vi "Configure Systems.vi"() -> ()   [LabVIEW 2009, in "POLARIS BME DG.lvlib" / "BME_DG_System.lvclass"]
uses:
  DG Classes/BME_DG_System/BME_DG_System.lvclass
  DetectDG.ctl
  System DG Selection.ctl
  LV-BME Interface/BME_DG_TriggerSettings.ctl
  LV-BME Interface/ClockSource.ctl
  SG08_Settings.ctl
  LV-BME Interface/BME_DG_V2TriggerSettings.ctl
  MSBusSignals.ctl
  LV-BME Interface/ChnlSettings.ctl
  Go_Done_Chnl_Settings.ctl
  GoSignalBits.ctl
  SG08_Chnl_Settings.ctl
  Chnl Settings Complete.ctl
  Card Config.ctl
  <vilib>/Utility/xml.llb/Write to XML File(array).vi
  DG Classes/BME_DG_Chnl/BME_DG_Chnl.lvclass
  POLARIS BME DG.lvlib
panel:
  out "Error?":bool
  in  "Build System":bool
  in  "ChnlToSwap":u16(ring) items=["a", "b", "c", "d", "e", "f", "ma", "mb", "mc", "md", "me", "mf", "sa", "sb", "sc", "sd", "se", "sf"]
  in  "SwapChnlWith":bool
  in  "Card2":u16(ring) caption="Swap with" items=["Master", "Master of Slave", "Slave of Master"]
  in  "SwapCardsWith":bool
  in  "Stop search":bool=TRUE
  in  "Find Chnl":u16(ring) items=["a", "b", "c", "d", "e", "f", "ma", "mb", "mc", "md", "me", "mf", "sa", "sb", "sc", "sd", "se", "sf"]
  in  "Find Card":u16(ring) items=["Master", "Master of Slave", "Slave of Master"]
  in  "stop":bool
  in  "Tab Control":T1(tab)=enum."Check"
  in  "InstalledDGs":T2[](array[typedef])
  in  "Select System":u16(ring) items=["Einsamer Master", "Master and Servant"]
  in  "Systems":T3[](array[typedef])
  in  "Selected DG":u16(ring) items=["0", "1", "2"]
  in  "Add":bool
  in  "Remove":bool
  in  "Empty Systems":bool
  in  "DetectDGs":bool
  in  "Card Config":T9(array[cluster]) {"Advanced Settings"."Trigger on MS Bus" format="%04x" items=["Local Primary0x1"=1, "Local Secondary0x2"=2, "Local Force 0x4"=4, "Resynchronize 0x8"=8, "StepBackOnBus 0x10"=16, "StartOnBus 0x20"=32, "InhibitOnBus 0x40"=64, "LoadDataOnBus 0x80"=128]; "Advanced Settings"."Force Trigger (µs)" min=0.0 format="%.6f"; "SG08_Settings"."StepBackTime (µs)" min=0.0 format="%.6f"; "SG08_Settings"."Gate Delay (µs)" format="%.3f"; "SG08_Settings"."Gate Level" min=-2.5 max=2.5 format="%.3g"; "Base Settings"."Gate Divider" min=1 max=1000000; "Base Settings"."Clock Source" items=["Internal Oscillator"=1, "External Trigger"=2, "Trigger-> Oscillator"=3, "MasterSlave Bus"=4]; "Base Settings"."Inhibit(µs)" format="%#_11g"}
  in  "Copy Chnl\n Names":bool=TRUE
  in  "Chnls":T14(array[cluster]) {"ChnParameter"."Delay (µs)" min=0.0 max=100000000.0 format="%.4f"; "G08_Chnl_Settings"."Pulse Width (µs)" min=0.0 max=8947840.0 format="%#.6f"; "Go and Done Signal"."Done Signal" format="%04x" items=["Local Primary"=1, "Local Secondary"=2, "Local Force"=4, "Master Primary"=16]; "Go and Done Signal"."Go Signal" format="%04x" items=["Local Primary0x1"=1, "Local Secondary0x2"=2, "Local Force 0x4"=4, "Resynchronize 0x8"=8, "Master Prim. 0x10"=16, "Master Sec. 0x20"=32, "Master Force  0x40"=64, "System Clock 0x80"=128, "Delay Clock 0x100"=256, "Inhibit Local 0x200"=512, "Start Local 0x400"=1024, "Start Bus 0x800"=2048, "Step Back Local 0x1000"=4096, "Step Back Bus 0x2000"=8192, "RunCircle 0x4000"=16384, "SyncReload 0x8000"=32768, "From E 0x10000"=65536, "From F 0x20000"=131072, "From Bus 0x40000"=262144]}
  in  "MS Signals Mask":u32 caption="Mask" format="%.0x"
  in  "MS Signals Bits to Mask":T8[](array[typedef]) format="%04x" items=["Local Primary0x1"=1, "Local Secondary0x2"=2, "Local Force 0x4"=4, "Resynchronize 0x8"=8, "StepBackOnBus 0x10"=16, "StartOnBus 0x20"=32, "InhibitOnBus 0x40"=64, "LoadDataOnBus 0x80"=128]
  in  "GoSignal Bits to Mask":T12[](array[typedef]) format="%04x" items=["Local Primary0x1"=1, "Local Secondary0x2"=2, "Local Force 0x4"=4, "Resynchronize 0x8"=8, "Master Prim. 0x10"=16, "Master Sec. 0x20"=32, "Master Force  0x40"=64, "System Clock 0x80"=128, "Delay Clock 0x100"=256, "Inhibit Local 0x200"=512, "Start Local 0x400"=1024, "Start Bus 0x800"=2048, "Step Back Local 0x1000"=4096, "Step Back Bus 0x2000"=8192, "RunCircle 0x4000"=16384, "SyncReload 0x8000"=32768, "From E 0x10000"=65536, "From F 0x20000"=131072, "From Bus 0x40000"=262144]
  in  "GoSignal Mask":u32 caption="Mask" format="%.0x"
  out "Problem Chnls out":string[](array[string])
  out "err and warnings":errorcluster[](array[cluster])
  out "Last Change":timestamp=timestamp(3422440183.453125 s since 1904-01-01)
  in  "Save":bool
  in  "Load":bool=TRUE
  in  "Config File":path
  # "DGNr"
  # "<=>"
  # "<=>"
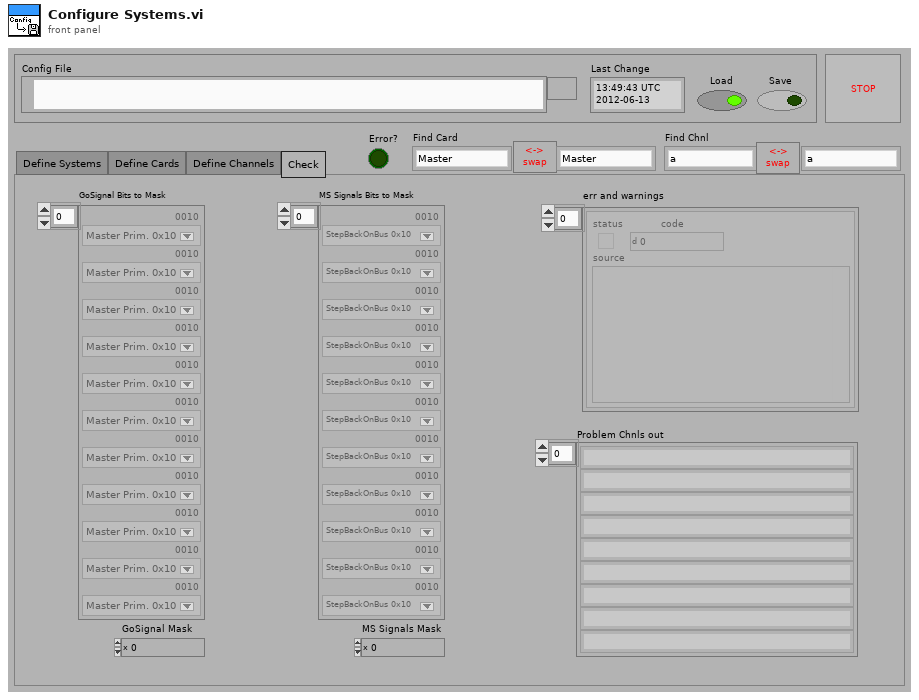
[diagram p1: front panel]
types:
  T1 = enum32{"Define Systems", "Define Cards", "Define Channels", "Check"}
  T2 = typedef "POLARIS BME DG.lvlib/DetectDG.ctl" = cluster{"DG_Number":i32, "DG_Product":i32, "Product Name":string, "Bus_Number":i32, "Slot_Number":i32, "Master":bool}
  T3 = typedef "POLARIS BME DG.lvlib/System DG Selection.ctl" = cluster{"Selected System DGs":T2[], "Name":string}
  T4 = typedef "POLARIS BME DG.lvlib/BME_DG_TriggerSettings.ctl" = cluster{"Clock Source":T5, " clock modulo":u32, "TriggerEnabled?":bool, "trigger modulo ":i32, "InputTerminated?":bool, "Inhibit(µs)":dbl, "TriggerLevel":dbl, "PresetValue":i32, "InternalTrigger?":bool, "InternalArm?":bool, "SWTrigger?":bool, "RisingEdge?":bool, "StopOnPreset?":bool, "ResetWhenDone?":bool, "Gate Divider":i32, "PositiveGate?":bool}
  T5 = typedef "POLARIS BME DG.lvlib/ClockSource.ctl" = i32
  T6 = typedef "POLARIS BME DG.lvlib/SG08_Settings.ctl" = cluster{"Gate Terminate":bool, "Gate Level":dbl, "Gate Delay (µs)":dbl, "StepBackTime (µs)":dbl, "Burst Counter":u32, "Trigger Divider":u32, "Trigger Multiplier":u32}
  T7 = typedef "POLARIS BME DG.lvlib/BME_DG_V2TriggerSettings.ctl" = cluster{"Trigger on MS Bus":T8, "Force Trigger (µs)":dbl, "Gate Type":bool, "Synchronize Gate":bool}
  T8 = typedef "POLARIS BME DG.lvlib/MSBusSignals.ctl" = u32
  T9 = cluster{"Logical Name":string, "Base Settings":T4, "SG08_Settings":T6, "Channel Names":string[], "Advanced Settings":T7}[]
  T10 = typedef "POLARIS BME DG.lvlib/ChnlSettings.ctl" = cluster{" Delay (µs)":dbl, "On?":bool, "PositiveVoltage?":bool, "50OhmTerminated? ":bool, "25OhmOutput?":bool}
  T11 = typedef "POLARIS BME DG.lvlib/Go_Done_Chnl_Settings.ctl" = cluster{"Go Signal":T12, "Done Signal":u32}
  T12 = typedef "POLARIS BME DG.lvlib/GoSignalBits.ctl" = u32
  T13 = typedef "POLARIS BME DG.lvlib/SG08_Chnl_Settings.ctl" = cluster{"Pulse Width (µs)":dbl, "Output Offset":u32, "Disconnect (E,F)":bool, "Onto MsBus (E,F)":bool, "Input Positive (E,F)":bool}
  T14 = cluster{"Channel Name":string, "ChnParameter":T10, "DelayFormula":string, "OutputModulo":i32, "Go and Done Signal":T11, "G08_Chnl_Settings":T13}[]
  T15 = typedef "POLARIS BME DG.lvlib/Chnl Settings Complete.ctl" = cluster{"Channel Name":string, "ChnParameter":T10, "DelayFormula":string, "OutputModulo":i32, "Go and Done Signal":T11, "G08_Chnl_Settings":T13}
  T16 = typedef "POLARIS BME DG.lvlib/Card Config.ctl" = cluster{"Logical Name":string, "Base Settings":T4, "SG08_Settings":T6, "Channel Names":string[], "Advanced Settings":T7}
  T17 = cluster{"Logical Name":string, "Base Settings":T4, "SG08_Settings":T6, "Channel Names":string[], "Advanced Settings":T7}
  T18 = cluster{"Channel Name":string, "ChnParameter":T10, "DelayFormula":string, "OutputModulo":i32, "Go and Done Signal":T11, "G08_Chnl_Settings":T13}
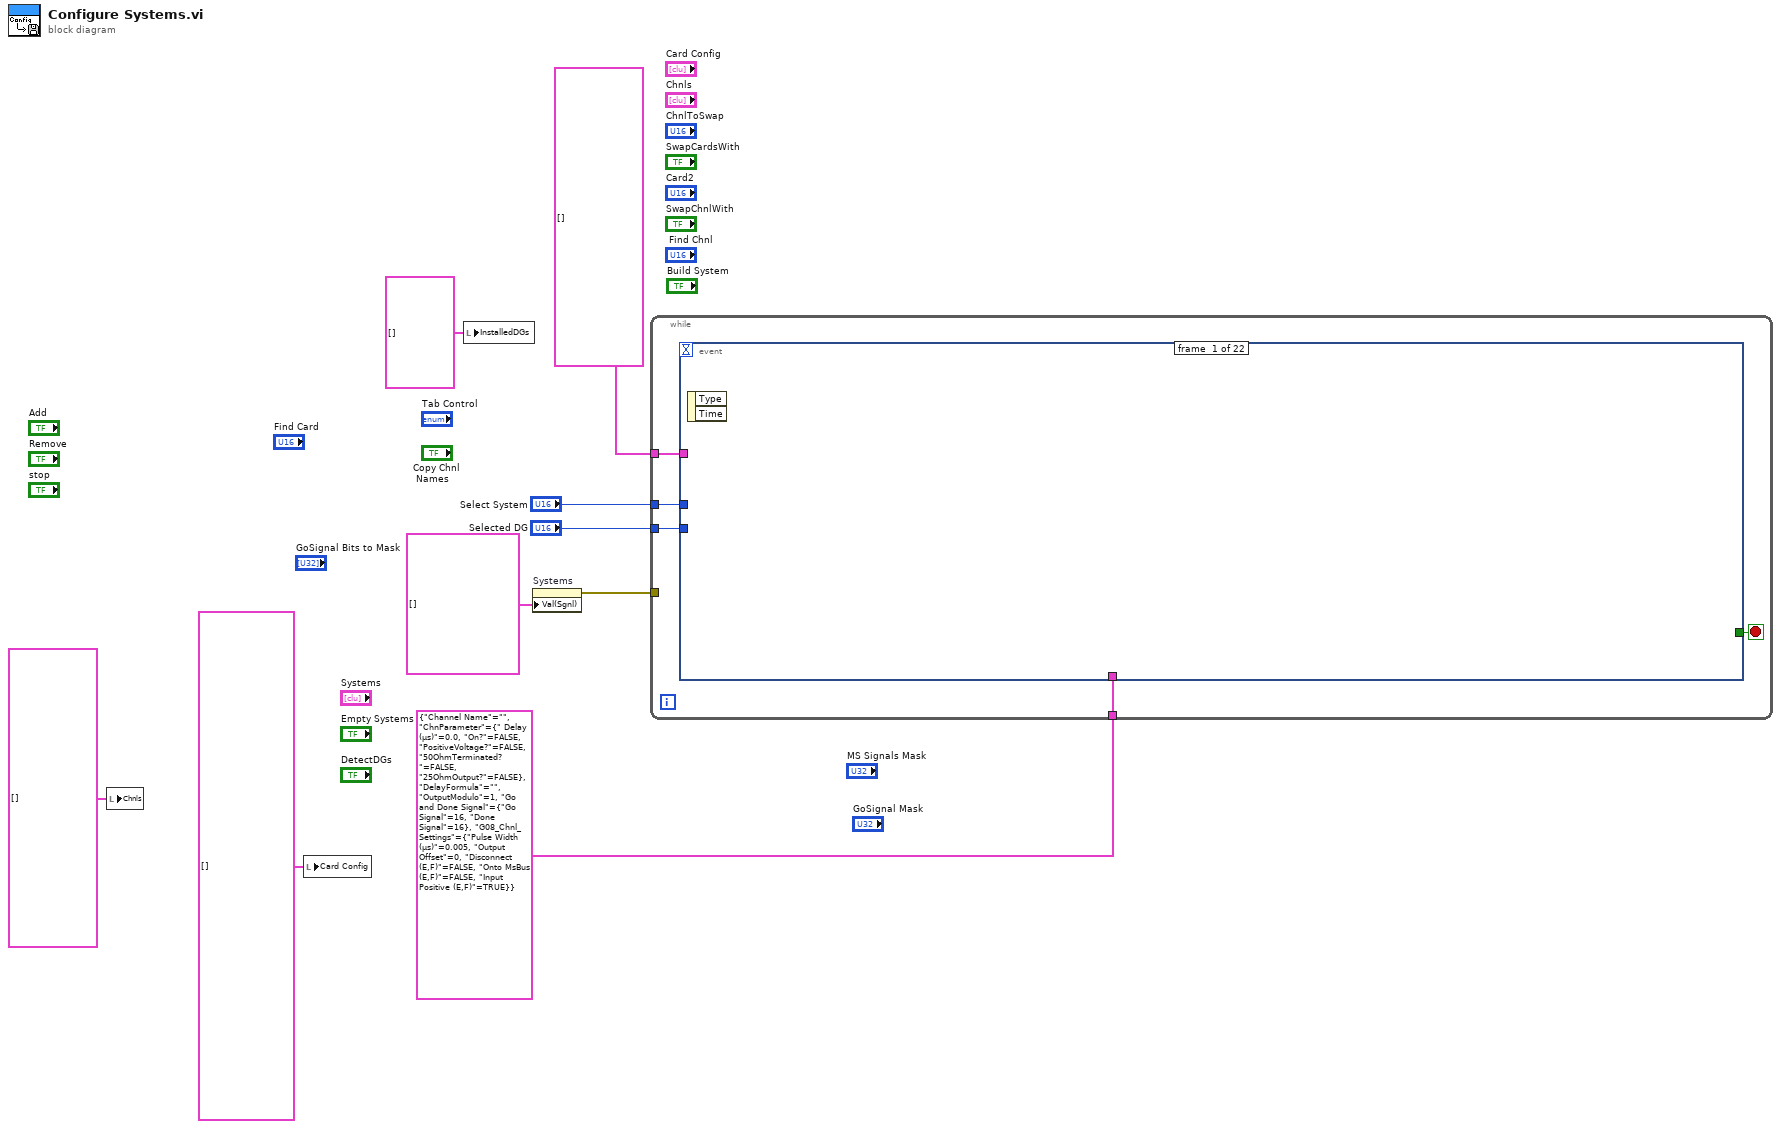
[diagram p0: block diagram]
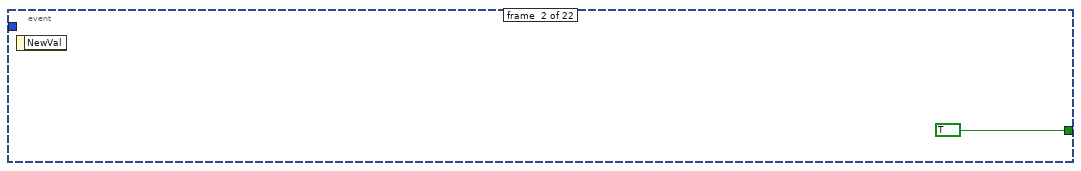
[diagram p2: hidden frame]
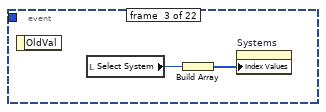
[diagram p3: hidden frame]
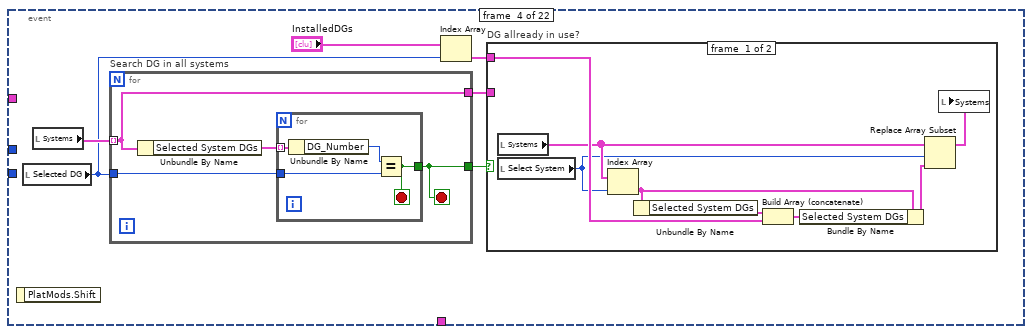
[diagram p4: hidden frame]
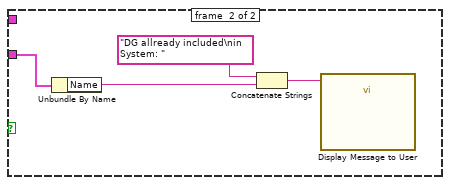
[diagram p5: hidden frame]
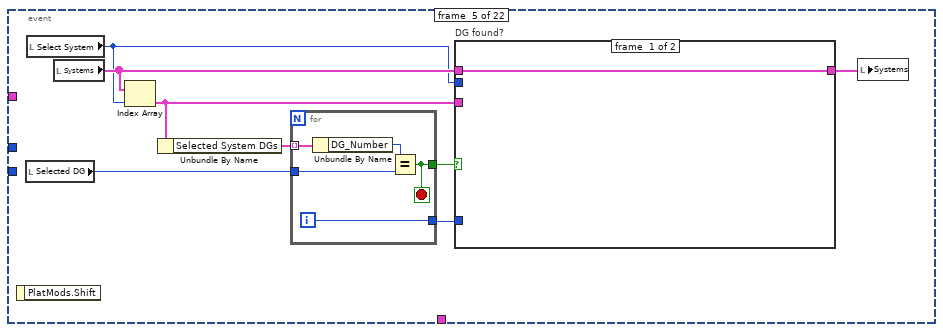
[diagram p6: hidden frame]
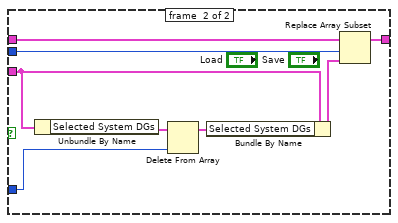
[diagram p7: hidden frame]
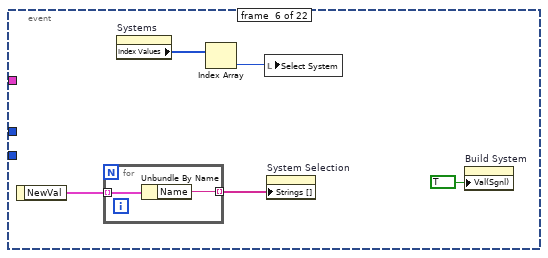
[diagram p8: hidden frame]
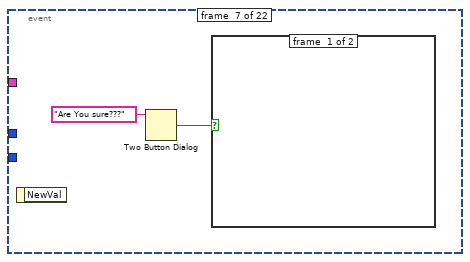
[diagram p9: hidden frame]
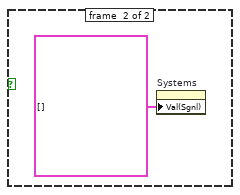
[diagram p10: hidden frame]
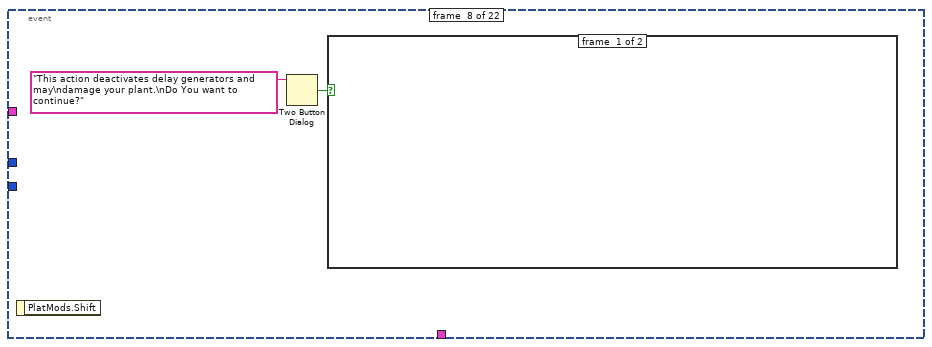
[diagram p11: hidden frame]
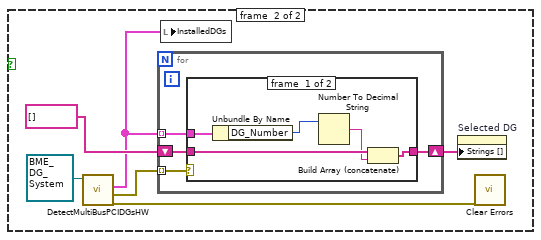
[diagram p12: hidden frame]
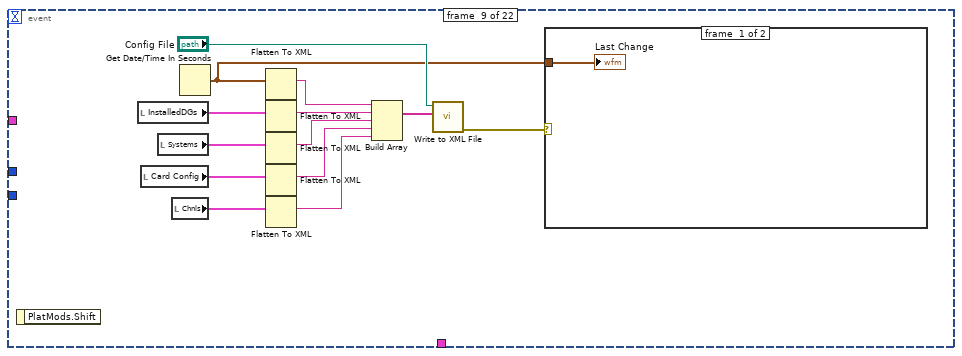
[diagram p14: hidden frame]
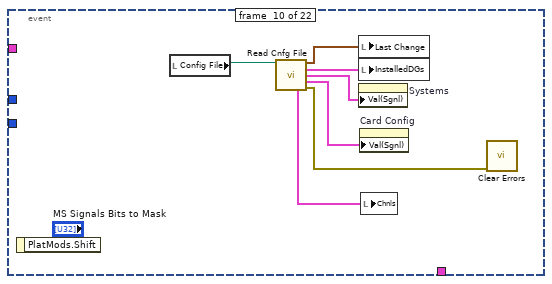
[diagram p16: hidden frame]
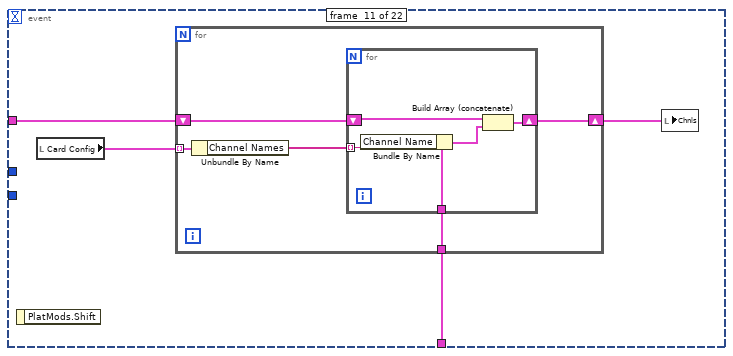
[diagram p17: hidden frame]
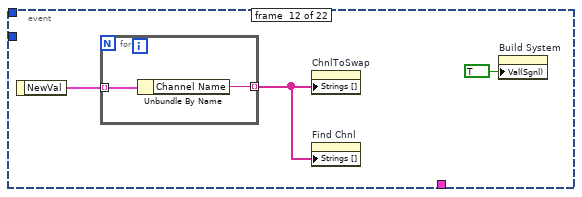
[diagram p18: hidden frame]
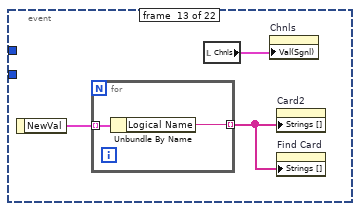
[diagram p19: hidden frame]
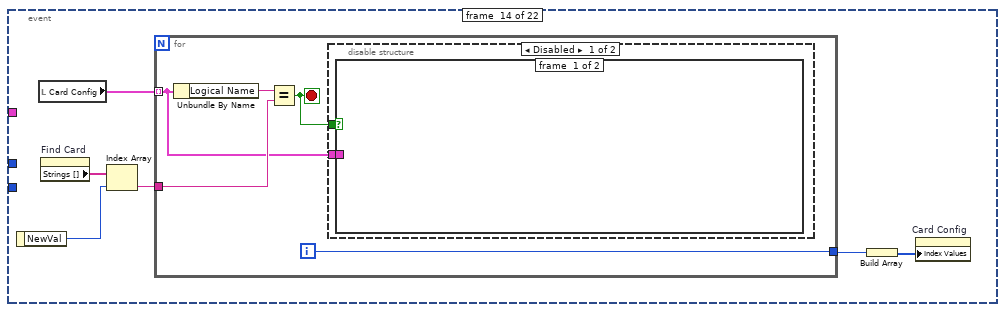
[diagram p20: hidden frame]
diagram:
  n1 = local write "Chnls"(T15[] [] ("Chnls")) -> ()
  n2 = local write "Card Config"(T16[] [] ("Card Config")) -> ()
  n3 = local write "InstalledDGs"(T2[] [] ("InstalledDGs")) -> ()
  n4 = property on="Systems" class="Arr (strict)"("Val(Sgnl)"=T3[] [] ("Value (Signaling)")) -> (error out=w6:errorcluster)  [unwired: 2 in, 1 out]
  n5 = while {
    tunnel: "Select System" -> [w13]
    tunnel: "Selected DG" -> [w12]
    tunnel: w6 -> [_]
    tunnel: T15 {"Channel Name"="", "ChnParameter"={" Delay (µs)"=0.0, "On?"=FALSE, "PositiveVoltage?"=FALSE, "50OhmTerminated? "=FALSE, "25OhmOutput?"=FALSE}, "DelayFormula"="", "OutputModulo"=1, "Go and Done Signal"={"Go Signal"=16, "Done Signal"=16}, "G08_Chnl_Settings"={"Pulse Width (µs)"=0.005, "Output Offset"=0, "Disconnect (E,F)"=FALSE, "Onto MsBus (E,F)"=FALSE, "Input Positive (E,F)"=TRUE}} ("Cluster") -> [w11]
    tunnel: T15[] [] -> [w10]
    stop <- w14 stop-if-true
    n6 = event shown="[11] \"Chnls\": Value Change" {
      selector: _ -> [_ _ _ _ _ _ _ _ _ _ _ _ _ _ _ _ _ _ _ _ _ _]
      dyn-events: _ -> [_ _ _ _ _ _ _ _ _ _ _ _ _ _ _ _ _ _ _ _ _ _]
      timeout: _ -> [_ _ _ _ _ _ _ _ _ _ _ _ _ _ _ _ _ _ _ _ _ _]
      tunnel: [_ TRUE _ _ _ _ _ _ _ _ _ _ _ _ _ _ _ _ _ _ _ _] -> w14
      tunnel: w13 -> [_ _ _ _ _ _ _ _ _ _ _ _ _ _ _ _ _ _ _ _ _ _]
      tunnel: w12 -> [_ _ _ _ _ _ _ _ _ _ _ _ _ _ _ _ _ _ _ _ _ _]
      tunnel: w11 -> [_ _ _ _ _ _ _ _ _ _ w116 _ _ _ _ _ _ _ _ _ _ _]
      tunnel: w10 -> [_ _ _ _ _ _ _ _ _ _ w115 _ _ _ _ _ _ _ _ _ _ _]
      event #0 {
        n7 = event-data() -> ()  [unwired: 1 in, 2 out]
      }
      event #1 {
        n8 = event-data() -> ()  [unwired: 1 in, 1 out]
      }
      event #2 {
        n9 = event-data() -> ()  [unwired: 1 in, 1 out]
        n10 = local read "Select System"() -> (w17:u16)
        n11 = Build Array(w17) -> (w16:u16[])
        n12 = property on="Systems" class="Arr (strict)"("Index Values"=w16) -> ()  [unwired: 2 in, 2 out]
      }
      event #3 {
        n13 = event-data() -> ()  [unwired: 1 in, 1 out]
        n14 = local read "Selected DG"() -> (w20:u16)
        n15 = local read "Systems"() -> (w23:T3[])
        n16 = for "Search DG in all systems" {
          tunnel: w23 -> [w36] mode=indexing
          tunnel: w20 -> [w38]
          tunnel: [w36] -> w21
          tunnel: [w37] -> w22
          stop <- w37 stop-if-true
          n17 = Unbundle By Name(w36) -> ("Selected System DGs"=w39:T2[])
          n18 = for {
            tunnel: w39 -> [w43] mode=indexing
            tunnel: w38 -> [w42]
            tunnel: [w40] -> w37
            stop <- w40 stop-if-true
            n19 = Unbundle By Name(w43) -> ("DG_Number"=w41:i32)
            n20 = Equal?(x=w41, y=w42) -> (x = y?=w40:bool)
          }
        }
        n21 = Index Array(array="InstalledDGs", index=w20) -> (element=w19:T2)
        n22 = case "DG allready in use?" shown="False" w22 {
          tunnel: w21 -> [_ w35]
          tunnel: w19 -> [w29 _]
          frame #0 {
            n23 = local read "Systems"() -> (w26:T3[])
            n24 = local read "Select System"() -> (w25:u16)
            n25 = Index Array(array=w26, index=w25) -> (element=w24:T3)
            n26 = Unbundle By Name(w24) -> ("Selected System DGs"=w31:T2[])
            n27 = Build Array (concatenate)(w31, w29) -> (w30:T2[])
            n28 = Bundle By Name(cluster=w24, "Selected System DGs"=w30) -> (w27:T3)
            n29 = Replace Array Subset(array=w26, new element=w27, index=w25) -> (w28:T3[])
            n30 = local write "Systems"(w28) -> ()
          }
          frame #1 {
            n31 = Unbundle By Name(w35) -> ("Name"=w32:string)
            n32 = Concatenate Strings("DG allready included\nin System: " ("string"), w32) -> (w34:string)
            n33 = call "Display Message to User"("Message"=w34) -> ()  [unwired: 9 in, 2 out]
          }
        }
      }
      event #4 {
        n34 = event-data() -> ()  [unwired: 1 in, 1 out]
        n35 = local read "Selected DG"() -> (w47:u16)
        n36 = local read "Select System"() -> (w44:u16)
        n37 = local read "Systems"() -> (w48:T3[])
        n38 = Index Array(array=w48, index=w44) -> (element=w45:T3)
        n39 = Unbundle By Name(w45) -> ("Selected System DGs"=w46:T2[])
        n40 = for {
          tunnel: w46 -> [w52] mode=indexing
          tunnel: w47 -> [w56]
          tunnel: [w55] -> w51
          tunnel: [w54] -> w50
          i -> [w54]
          stop <- w55 stop-if-true
          n41 = Unbundle By Name(w52) -> ("DG_Number"=w53:i32)
          n42 = Equal?(x=w53, y=w56) -> (x = y?=w55:bool)
        }
        n43 = case "DG found?" shown="True" w51 {
          tunnel: w50 -> [_ w62]
          tunnel: w48 -> [w57 w65]
          tunnel: [w57 w64] -> w49
          tunnel: w45 -> [_ w61]
          tunnel: w44 -> [_ w58]
          frame #0 {
          }
          frame #1 {
            n44 = Unbundle By Name(w61) -> ("Selected System DGs"=w63:T2[])
            n45 = Delete From Array(array=w63, index=w62) -> (array with subset deleted=w60:T2[])  [unwired: 1 in, 1 out]
            n46 = Bundle By Name(cluster=w61, "Selected System DGs"=w60) -> (w59:T3)
            n47 = Replace Array Subset(array=w65, new element=w59, index=w58) -> (w64:T3[])
          }
        }
        n48 = local write "Systems"(w49) -> ()
      }
      event #5 {
        n49 = event-data() -> ("NewVal"=w70:T3[])  [unwired: 1 in]
        n50 = for {
          tunnel: w70 -> [w72] mode=indexing
          tunnel: [w71] -> w69 mode=indexing
          n51 = Unbundle By Name(w72) -> ("Name"=w71:string)
        }
        n52 = property on="Systems" class="Arr (strict)"() -> ("Index Values"=w68:u32[])  [unwired: 2 in, 2 out]
        n53 = Index Array(array=w68) -> (element=w67:u32)  [unwired: 1 in]
        n54 = local write "Select System"(w67) -> ()
        n55 = property on="System Selection" class="Ring (strict)"("Strings []"=w69) -> ()  [unwired: 2 in, 2 out]
        n56 = property on="Build System" class="Bool (strict)"("Val(Sgnl)"=TRUE ("Value (Signaling)")) -> ()  [unwired: 2 in, 2 out]
      }
      event #6 {
        n57 = event-data() -> ()  [unwired: 1 in, 1 out]
        n58 = Two Button Dialog(message="Are You sure???") -> (T button?=w73:bool)  [unwired: 2 in]
        n59 = case shown="True" w73 {
          frame #0 {
          }
          frame #1 {
            n60 = property on="Systems" class="Arr (strict)"("Val(Sgnl)"=T3[] [] ("Value (Signaling)")) -> ()  [unwired: 2 in, 2 out]
          }
        }
      }
      event #7 {
        n61 = event-data() -> ()  [unwired: 1 in, 1 out]
        n62 = Two Button Dialog(message="This action deactivates delay generators and may\ndamage your plant.\nDo You want to continue?") -> (T button?=w76:bool)  [unwired: 2 in]
        n63 = case shown="True" w76 {
          frame #0 {
          }
          frame #1 {
            n64 = call "DetectMultiBusPCIDGsHW.vi"("BME_DG_System in"=refnum<class "BME_DG_System.lvclass"> refnum) -> ("error out"=w78:errorcluster, "Errors"=w81:errorcluster[], "InstalledDGs"=w79:T2[])  [unwired: 6 in, 2 out]
            n65 = for {
              tunnel: w81 -> [w84] mode=indexing
              tunnel: w79 -> [w86] mode=indexing
              shift-right: [w87] -> w82
              shift-left: string[] [] -> [w85]
              n66 = case shown="No Error" w84 {
                tunnel: [w92 w93] -> w87
                tunnel: w86 -> [w90 _]
                tunnel: w85 -> [w91 w93]
                frame #0 {
                  n67 = Unbundle By Name(w90) -> ("DG_Number"=w89:i32)
                  n68 = Number To Decimal String(number=w89) -> (decimal integer string=w88:string)  [unwired: 1 in]
                  n69 = Build Array (concatenate)(w91, w88) -> (w92:string[])
                }
                frame #1 {
                }
              }
            }
            n70 = local write "InstalledDGs"(w79) -> ()
            n71 = property on="Selected DG" class="Ring (strict)"("Strings []"=w82) -> ()  [unwired: 2 in, 2 out]
            n72 = call <vilib>:"Clear Errors.vi"("error in (no error)"=w78) -> ()  [unwired: 6 in, 1 out]
          }
        }
      }
      event #8 {
        n73 = event-data() -> ()  [unwired: 1 in, 1 out]
        n74 = local read "InstalledDGs"() -> (w106:T2[])
        n75 = local read "Card Config"() -> (w97:T9)
        n76 = local read "Systems"() -> (w105:T3[])
        n77 = local read "Chnls"() -> (w95:T14)
        n78 = Get Date/Time In Seconds() -> (seconds since 1Jan1904=w99:timestamp)
        n79 = Flatten To XML(anything=w99) -> (xml string=w104:string)
        n80 = Flatten To XML(anything=w106) -> (xml string=w103:string)
        n81 = Flatten To XML(anything=w105) -> (xml string=w102:string)
        n82 = Flatten To XML(anything=w97) -> (xml string=w96:string)
        n83 = Flatten To XML(anything=w95) -> (xml string=w94:string)
        n84 = Build Array(w104, w103, w102, w96, w94) -> (w101:string[])
        n85 = call-poly <vilib>:"Write to XML File.vi"("XML Input"=w101, "XML File Path"="Config File") -> ("error out"=w98:errorcluster)  [unwired: 7 in, 2 out]
        n86 = case shown="Error" w98 {
          tunnel: w99 -> [w107 _]
          frame #0 {
            "Last Change" <- w107
          }
          frame #1 {
          }
        }
      }
      event #9 {
        n87 = event-data() -> ()  [unwired: 1 in, 1 out]
        n88 = local read "Config File"() -> (w114:path)
        n89 = call "Read Cnfg File.vi"("Config File"=w114) -> ("Last Change"=w113:timestamp, "InstalledDGs"=w112:T2[], "DGSystems"=w111:T3[], "Cards"=w110:T16[], "Chnls"=w109:T15[], "error out"=w108:errorcluster)  [unwired: 9 in]
        n90 = local write "Last Change"(w113) -> ()
        n91 = local write "InstalledDGs"(w112) -> ()
        n92 = property on="Systems" class="Arr (strict)"("Val(Sgnl)"=w111) -> ()  [unwired: 2 in, 2 out]
        n93 = property on="Card Config" class="Arr (strict)"("Val(Sgnl)"=w110) -> ()  [unwired: 2 in, 2 out]
        n94 = local write "Chnls"(w109) -> ()
        n95 = call <vilib>:"Clear Errors.vi"("error in (no error)"=w108) -> ()  [unwired: 6 in, 1 out]
      }
      event #10 {
        n96 = event-data() -> ()  [unwired: 1 in, 1 out]
        n97 = local read "Card Config"() -> (w118:T9)
        n98 = for {
          tunnel: w118 -> [w123] mode=indexing
          shift-right: [w120] -> w117
          shift-left: w115 -> [w121]
          tunnel: w116 -> [w119]
          n99 = Unbundle By Name(w123) -> ("Channel Names"=w122:string[])
          n100 = for {
            tunnel: w122 -> [w125] mode=indexing
            shift-right: [w127] -> w120
            shift-left: w121 -> [w128]
            tunnel: w119 -> [w126]
            n101 = Bundle By Name(cluster=w126, "Channel Name"=w125) -> (w124:T15)
            n102 = Build Array (concatenate)(w128, w124) -> (w127:T15[])
          }
        }
        n103 = local write "Chnls"(w117) -> ()
      }
      event #11 {
        n104 = event-data() -> ("NewVal"=w131:T14)  [unwired: 1 in]
        n105 = for {
          tunnel: w131 -> [w132] mode=indexing
          tunnel: [w133] -> w130 mode=indexing
          n106 = Unbundle By Name(w132) -> ("Channel Name"=w133:string)
        }
        n107 = property on="ChnlToSwap" class="Ring (strict)"("Strings []"=w130) -> ()  [unwired: 2 in, 2 out]
        n108 = property on="Find Chnl" class="Ring (strict)"("Strings []"=w130) -> ()  [unwired: 2 in, 2 out]
        n109 = property on="Build System" class="Bool (strict)"("Val(Sgnl)"=TRUE ("Value (Signaling)")) -> ()  [unwired: 2 in, 2 out]
      }
      event #12 {
        n110 = event-data() -> ("NewVal"=w136:T9)  [unwired: 1 in]
        n111 = for {
          tunnel: w136 -> [w138] mode=indexing
          tunnel: [w137] -> w135 mode=indexing
          n112 = Unbundle By Name(w138) -> ("Logical Name"=w137:string)
        }
        n113 = local read "Chnls"() -> (w134:T14)
        n114 = property on="Chnls" class="Arr (strict)"("Val(Sgnl)"=w134) -> ()  [unwired: 2 in, 2 out]
        n115 = property on="Card2" class="Ring (strict)"("Strings []"=w135) -> ()  [unwired: 2 in, 2 out]
        n116 = property on="Find Card" class="Ring (strict)"("Strings []"=w135) -> ()  [unwired: 2 in, 2 out]
      }
      event #13 {
        n117 = event-data() -> ("NewVal"=w140:u16)  [unwired: 1 in]
        n118 = local read "Card Config"() -> (w142:T9)
        n119 = property on="Find Card" class="Ring (strict)"() -> ("Strings []"=w141:string[])  [unwired: 2 in, 2 out]
        n120 = Index Array(array=w141, index=w140) -> (element=w143:string)
        n121 = for {
          tunnel: w142 -> [w145] mode=indexing
          tunnel: w143 -> [w148]
          tunnel: [w147] -> w144
          i -> [w147]
          stop <- w146 stop-if-true
          n122 = Unbundle By Name(w145) -> ("Logical Name"=w149:string)
          n123 = Equal?(x=w149, y=w148) -> (x = y?=w146:bool)
          n124 = disable-structure shown="Disabled" {
            disable-tunnel: w146 -> [w151 _]
            disable-tunnel: w145 -> [w150 _]
            frame #0 {
              n125 = case shown="True" w151 {
                tunnel: w150 -> [_ w154]
                frame #0 {
                }
                frame #1 {
                  n126 = Unbundle By Name(w154) -> ("Channel Names"=w153:string[])
                  n127 = property on="Find Chnl" class="Ring (strict)"() -> ("Strings []"=w155:string[])  [unwired: 2 in, 2 out]
                  n128 = Index Array(array=w153) -> (element=w152:string)  [unwired: 1 in]
                  n129 = for {
                    tunnel: w155 -> [w159] mode=indexing
                    tunnel: w152 -> [w158]
                    i -> [w156]
                    stop <- w157 stop-if-true
                    n130 = Equal?(x=w159, y=w158) -> (x = y?=w157:bool)
                    n131 = case shown="True" w157 {
                      selector: w157 -> [_ w160]
                      tunnel: w156 -> [_ w161]
                      frame #0 {
                      }
                      frame #1 {
                        n132 = local write "Stop search"(w160) -> ()
                        n133 = property on="Find Chnl" class="Ring (strict)"("Val(Sgnl)"=w161) -> ()  [unwired: 2 in, 2 out]
                      }
                    }
                  }
                }
              }
            }
            frame #1 {
            }
          }
        }
        n134 = Build Array(w144) -> (w139:i32[])
        n135 = property on="Card Config" class="Arr (strict)"("Index Values"=w139) -> ()  [unwired: 2 in, 2 out]
      }
      event #14 {
        n136 = event-data() -> ("NewVal"=w172:u16)  [unwired: 1 in]
        n137 = local read "Card Config"() -> (w173:T9)
        n138 = property on="Find Chnl" class="Ring (strict)"() -> ("Strings []"=w171:string[])  [unwired: 2 in, 2 out]
        n139 = Index Array(array=w171, index=w172) -> (element=w166:string)
        n140 = for {
          tunnel: w173 -> [w187] mode=indexing
          tunnel: w166 -> [w185]
          tunnel: [w184] -> w170
          tunnel: [w183] -> w169
          i -> [w184]
          stop <- w183 stop-if-true
          n141 = Unbundle By Name(w187) -> ("Channel Names"=w186:string[])
          n142 = for {
            tunnel: w186 -> [w189] mode=indexing
            tunnel: w185 -> [w190]
            tunnel: [w188] -> w183
            stop <- w188 stop-if-true
            n143 = Equal?(x=w189, y=w190) -> (x = y?=w188:bool)
          }
        }
        n144 = Not(x="Stop search") -> (.not. x?=w162:bool)
        n145 = And(x=w169, y=w162) -> (x .and. y?=w164:bool)
        n146 = local read "Chnls"() -> (w168:T14)
        n147 = case shown="True" w164 {
          tunnel: w170 -> [_ w182]
          frame #0 {
            n148 = local write "Stop search"(FALSE ("Stop search")) -> ()
          }
          frame #1 {
            n149 = property on="Find Card" class="Ring (strict)"("Val(Sgnl)"=w182) -> ()  [unwired: 2 in, 2 out]
          }
        }
        n150 = for {
          tunnel: w168 -> [w180] mode=indexing
          tunnel: w166 -> [w178]
          tunnel: [w177] -> w167
          tunnel: [w176] -> w165
          i -> [w177]
          stop <- w176 stop-if-true
          n151 = Unbundle By Name(w180) -> ("Channel Name"=w179:string)
          n152 = Equal?(x=w178, y=w179) -> (x = y?=w176:bool)
        }
        n153 = case shown="True" w165 {
          tunnel: w167 -> [_ w174]
          frame #0 {
          }
          frame #1 {
            n154 = Build Array(w174) -> (w175:i32[])
            n155 = property on="Chnls" class="Arr (strict)"("Index Values"=w175) -> ()  [unwired: 2 in, 2 out]
          }
        }
      }
      event #15 {
        n156 = event-data() -> ("NewVal"=w193:T12[])  [unwired: 1 in]
        n157 = for {
          tunnel: w193 -> [w196] mode=indexing
          shift-right: [w195] -> w191
          shift-left: 0 -> [w194]
          n158 = Or(x=w194, y=w196) -> (x .or. y?=w195:T12)
        }
        n159 = local write "GoSignal Mask"(w191) -> ()
      }
      event #16 {
        n160 = event-data() -> ("NewVal"=w199:T8[])  [unwired: 1 in]
        n161 = for {
          tunnel: w199 -> [w202] mode=indexing
          shift-right: [w201] -> w197
          shift-left: 0 -> [w200]
          n162 = Or(x=w200, y=w202) -> (x .or. y?=w201:T8)
        }
        n163 = local write "MS Signals Mask"(w197) -> ()
      }
      event #17 {
        n164 = event-data() -> ("NewVal"=w203:bool)  [unwired: 1 in]
        n165 = case shown="True" w203 {
          frame #0 {
          }
          frame #1 {
            n166 = local read "Card Config"() -> (w210:T9)
            n167 = local read "Find Card"() -> (w208:u16)
            n168 = local read "Card2"() -> (w205:u16)
            n169 = Index Array(array=w210, index #1=w208, index #2=w205) -> (element #1=w206:T17, element #2=w207:T17)
            n170 = Replace Array Subset(array=w210, new element=w207, index=w208) -> (w209:T9)
            n171 = Replace Array Subset(array=w209, new element=w206, index=w205) -> (w204:T9)
            n172 = property on="Card Config" class="Arr (strict)"("Val(Sgnl)"=w204) -> ()  [unwired: 2 in, 2 out]
          }
        }
      }
      event #18 {
        n173 = event-data() -> ()  [unwired: 1 in, 2 out]
        n174 = local read "Chnls"() -> (w213:T14)
        n175 = local read "Find Chnl"() -> (w212:u16)
        n176 = local read "ChnlToSwap"() -> (w211:u16)
        n177 = Index Array(array=w213, index #1=w212, index #2=w211) -> (element #1=w215:T18, element #2=w216:T18)
        n178 = Replace Array Subset(array=w213, new element=w216, index=w212) -> (w217:T14)
        n179 = Replace Array Subset(array=w217, new element=w215, index=w211) -> (w214:T14)
        n180 = property on="Chnls" class="Arr (strict)"("Val(Sgnl)"=w214) -> ()  [unwired: 2 in, 2 out]
      }
      event #19 {
        n181 = event-data() -> ("NewVal"=w221:u32)  [unwired: 1 in]
        n182 = Number To Boolean Array(number=w221) -> (Boolean array=w220:bool[])
        n183 = for {
          tunnel: w220 -> [w225] mode=indexing
          shift-right: [w222] -> w218
          shift-left: i32[] [] ("Array") -> [w223]
          i -> [w224]
          n184 = case shown="True" w225 {
            tunnel: w224 -> [_ w230]
            tunnel: w223 -> [w226 w228]
            tunnel: [w226 w227] -> w222
            frame #0 {
            }
            frame #1 {
              n185 = Logical Shift(y=w230, x=1) -> (x << y=w229:i32)
              n186 = Build Array (concatenate)(w228, w229) -> (w227:i32[])
            }
          }
        }
        n187 = local write "GoSignal Bits to Mask"(w218) -> ()
      }
      event #20 {
        n188 = event-data() -> ("NewVal"=w235:u32)  [unwired: 1 in]
        n189 = Number To Boolean Array(number=w235) -> (Boolean array=w234:bool[])
        n190 = for {
          tunnel: w234 -> [w239] mode=indexing
          shift-right: [w236] -> w232
          shift-left: i32[] [] ("Array") -> [w237]
          i -> [w238]
          n191 = case shown="True" w239 {
            tunnel: w238 -> [_ w244]
            tunnel: w237 -> [w240 w242]
            tunnel: [w240 w241] -> w236
            frame #0 {
            }
            frame #1 {
              n192 = Logical Shift(y=w244, x=1) -> (x << y=w243:i32)
              n193 = Build Array (concatenate)(w242, w243) -> (w241:i32[])
            }
          }
        }
        n194 = local write "MS Signals Bits to Mask"(w232) -> ()
      }
      event #21 {
        n195 = event-data() -> ("NewVal"=w246:bool)  [unwired: 1 in]
        n196 = case shown="True" w246 {
          frame #0 {
          }
          frame #1 {
            n197 = local read "Card Config"() -> (w258:T9)
            n198 = local read "Systems"() -> (w259:T3[])
            n199 = local read "Chnls"() -> (w254:T14)
            n200 = for {
              tunnel: [w282] -> w255 mode=indexing
              tunnel: [w281] -> w253
              tunnel: w259 -> [w280] mode=indexing
              tunnel: w258 -> [w279]
              tunnel: w254 -> [w278]
              tunnel: [w277] -> w249 mode=indexing
              tunnel: refnum<class "BME_DG_System.lvclass"> refnum ("BME_DG_System in") -> [w276]
              n201 = call "InitDGSystem and HW.vi"("InitHW(false)"=FALSE ("InitHW(True)"), "System"=w280, "Chnls"=w278, "Cards"=w279, "BME_DG_System in"=w276) -> ("error out"=w277:errorcluster, "Problem Chnls out"=w281:string[], "BME_DG_System in"=w282:refnum<class "BME_DG_System.lvclass">)  [unwired: 4 in]
            }
            n202 = for "Show Abs Delayvalues" {
              tunnel: w254 -> [w266] mode=indexing
              tunnel: [w264] -> w256 mode=indexing
              tunnel: w255 -> [w270]
              tunnel: [w263] -> w251 mode=indexing
              shift-right: [w261] -> w252
              shift-left: w253 -> [w262]
              n203 = Unbundle By Name(w266) -> ("Channel Name"=w260:string)
              n204 = call "Select System By Chnl.vi"("ChnlName"=w260, "SystemsIn"=w270) -> ("error out"=w269:errorcluster, "BME_DG_Chnl"=w268:refnum<class "BME_DG_Chnl.lvclass">)  [unwired: 5 in, 3 out]
              n205 = call-dynamic "Read ChnParameter.vi"("error in (no error)"=w269, "BME_DG_Chnl in"=w268) -> ("error out"=w263:errorcluster, "ChnParemater"=w267:T10)  [unwired: 4 in, 4 out]
              n206 = Unbundle By Name(w267) -> ("Delay (µs)"=w265:dbl)
              n207 = case shown="Error" w263 {
                tunnel: w262 -> [w271 w274]
                tunnel: [w271 w273] -> w261
                tunnel: w260 -> [_ w272]
                frame #0 {
                }
                frame #1 {
                  n208 = Build Array (concatenate)(w274, w272) -> (w273:string[])
                }
              }
              n209 = Bundle By Name(cluster=w266, "ChnParameter.Delay (µs)"=w265) -> (w264:T18)
            }
            "Problem Chnls out" <- w252
            n210 = local write "Chnls"(w256) -> ()
            n211 = Build Array (concatenate)(w251, w249) -> (w250:errorcluster[])
            n212 = call "Remove empty Errors.vi"("all error clusters"=w250) -> ("err and warnings"=→"err and warnings":errorcluster[], "some problems?"=→"Error?":bool)  [unwired: 9 in]
          }
        }
      }
    }
  }
